vi "Create Statement Line.vi"(6 "Delimiter":string=", ", 8 "Error In":errorcluster, 11 "Statement":T1) -> (0 "Error Out":errorcluster, 3 "Line":string)   [LabVIEW 2018, in "Toolkit.lvlib"]
doc: "Converts a logging statement to a Comma Separated Values (CSV) line."
uses:
  Toolkit.lvlib
  Type Definitions/Statement.ctl
  Type Definitions/Tag.ctl
  <vilib>/dlg_ctls.llb/Space Constant.vi
  <vilib>/Utility/error.llb/Trim Whitespace.vi
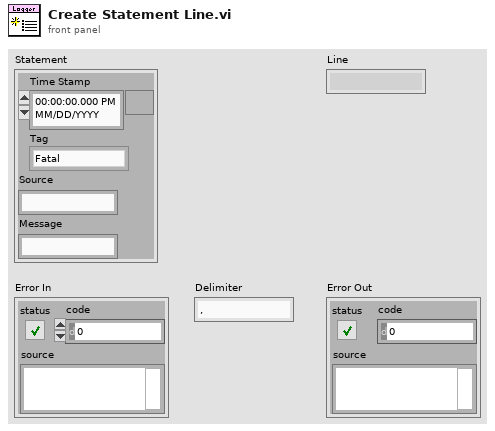
[diagram p1: front panel]
types:
  T1 = typedef "Toolkit.lvlib/Statement.ctl" = cluster{"Time Stamp":timestamp, "Tag":T2, "Source":string, "Message":string}
  T2 = typedef "Toolkit.lvlib/Tag.ctl" = enum16{"Fatal", "Error", "Warn", "Info", "Debug", "Trace"}
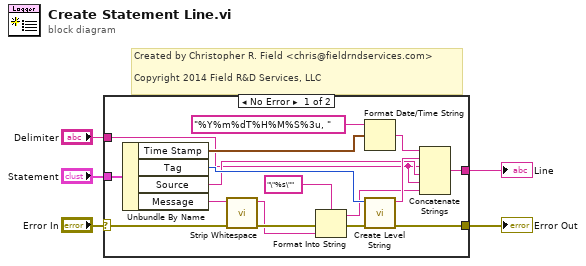
[diagram p0: block diagram]
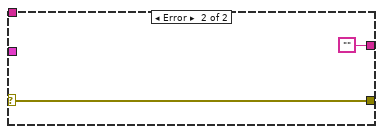
[diagram p2: hidden frame]
diagram:
  # "Created by Christopher R. Field <chris@fieldrndservices.com>\n\nCopyright 2014 Field R&D Services, LLC"
  n1 = case shown="No Error" "Error In" {
    selector: "Error In" -> [w13 w24]
    tunnel: "Statement" -> [w22 _]
    tunnel: [w15 w24] -> w3
    tunnel: [w14 ""] -> w2
    tunnel: "Delimiter" -> [w6 _]
    frame No Error {
      n2 = Unbundle By Name(w22) -> ("Time Stamp"=w21:timestamp, "Tag"=w19:T2, "Source"=w16:string, "Message"=w11:string)
      n3 = call "Strip Whitespace.vi"("Error In"=w13, "Text"=w11) -> ("Error Out"=w12:errorcluster, "Stripped Text"=w8:string)  [unwired: 8 in]
      n4 = Format Into String(format string="\"%s\"", error in=w12, w8) -> (resulting string=w7:string, error out=w10:errorcluster)  [unwired: 1 in]
      n5 = Format Date/Time String(time format string (%c)="%Y%m%dT%H%M%S%3u, ", seconds (now)=w21) -> (date/time string=w18:string)  [unwired: 1 in]
      n6 = call "Create Level String.vi"("Error In"=w10, "Level"=w19) -> ("Error Out"=w15:errorcluster, "String"=w17:string)  [unwired: 8 in]
      n7 = Concatenate Strings(w18, w17, w6, w16, w6, w7) -> (w14:string)
    }
    frame Error {
    }
  }
  "Error Out" <- w3
  "Line" <- w2
